vi "hvaccuid.vi"(3 "ID":i32) -> (0 "Temp id":i32, 1 "Volt id":i32)   [LabVIEW 2017]
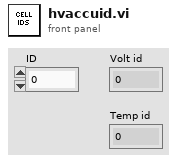
[diagram p1: front panel]
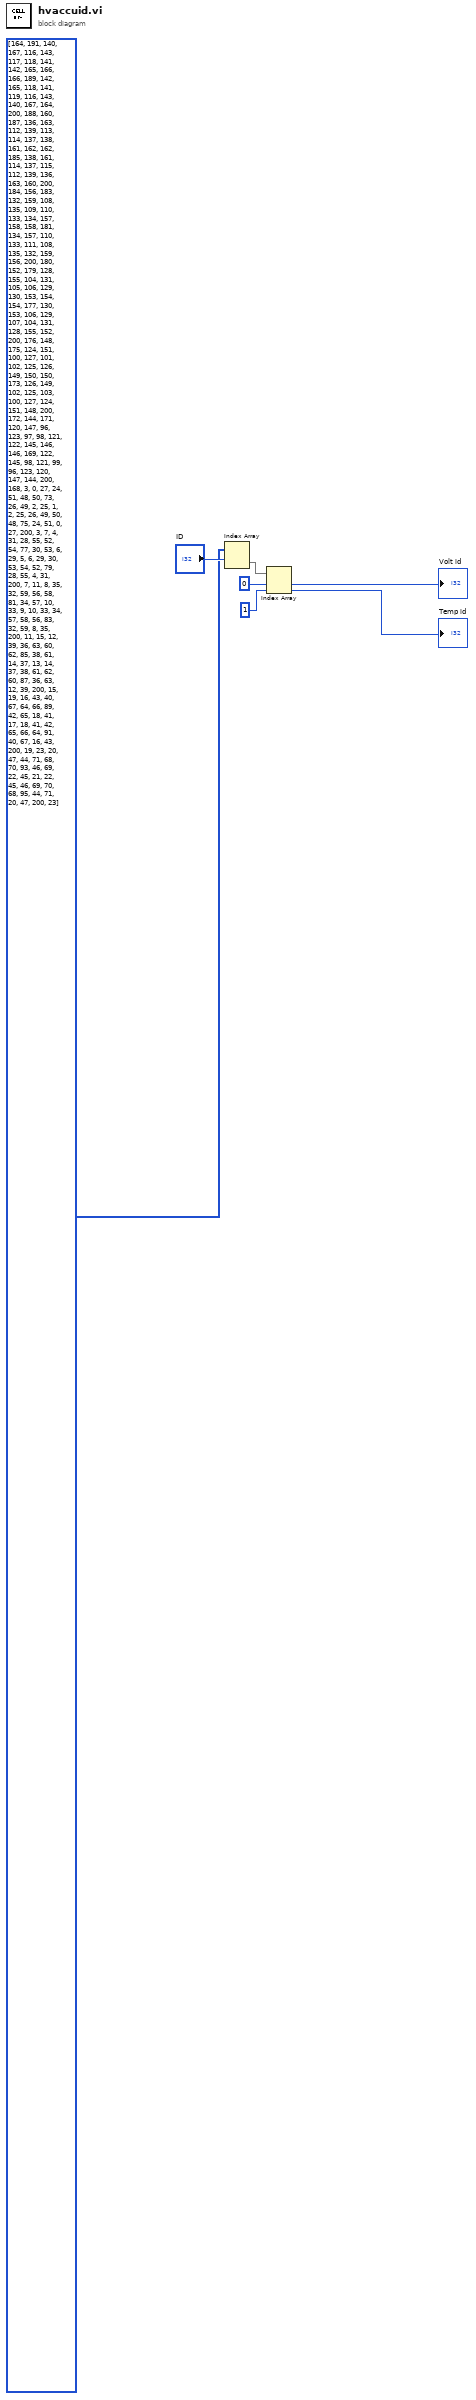
[diagram p0: block diagram]
diagram:
  n1 = Index Array(array=i32[][] [[164, 191], [140, 167], [116, 143], [117, 118], [141, 142], [165, 166], [166, 189], [142, 165], [118, 141], [119, 116], [143, 140], [167, 164], [200, 188], [160, 187], [136, 163], [112, 139], [113, 114], [137, 138], [161, 162], [162, 185], [138, 161], [114, 137], [115, 112], [139, 136], [163, 160], [200, 184], [156, 183], [132, 159], [108, 135], [109, 110], [133, 134], [157, 158], [158, 181], [134, 157], [110, 133], [111, 108], [135, 132], [159, 156], [200, 180], [152, 179], [128, 155], [104, 131], [105, 106], [129, 130], [153, 154], [154, 177], [130, 153], [106, 129], [107, 104], [131, 128], [155, 152], [200, 176], [148, 175], [124, 151], [100, 127], [101, 102], [125, 126], [149, 150], [150, 173], [126, 149], [102, 125], [103, 100], [127, 124], [151, 148], [200, 172], [144, 171], [120, 147], [96, 123], [97, 98], [121, 122], [145, 146], [146, 169], [122, 145], [98, 121], [99, 96], [123, 120], [147, 144], [200, 168], [3, 0], [27, 24], [51, 48], [50, 73], [26, 49], [2, 25], [1, 2], [25, 26], [49, 50], [48, 75], [24, 51], [0, 27], [200, 3], [7, 4], [31, 28], [55, 52], [54, 77], [30, 53], [6, 29], [5, 6], [29, 30], [53, 54], [52, 79], [28, 55], [4, 31], [200, 7], [11, 8], [35, 32], [59, 56], [58, 81], [34, 57], [10, 33], [9, 10], [33, 34], [57, 58], [56, 83], [32, 59], [8, 35], [200, 11], [15, 12], [39, 36], [63, 60], [62, 85], [38, 61], [14, 37], [13, 14], [37, 38], [61, 62], [60, 87], [36, 63], [12, 39], [200, 15], [19, 16], [43, 40], [67, 64], [66, 89], [42, 65], [18, 41], [17, 18], [41, 42], [65, 66], [64, 91], [40, 67], [16, 43], [200, 19], [23, 20], [47, 44], [71, 68], [70, 93], [46, 69], [22, 45], [21, 22], [45, 46], [69, 70], [68, 95], [44, 71], [20, 47], [200, 23]], index (row)="ID") -> (element=w1:i32[])  [unwired: 1 in]
  n2 = Index Array(array=w1, index #1=0 ("index"), index #2=1 ("index")) -> (element #1=→"Volt id":i32, element #2=→"Temp id":i32)
